vi "stop watch (1).vi"() -> ()   [LabVIEW 2016]
panel:
  out "start time":timestamp
  out "Started":bool
  in  "OK Button":bool
  out "Elapsed time (seconds)":dbl
  in  "stop":bool
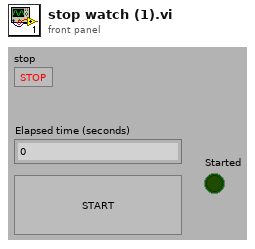
[diagram p1: front panel]
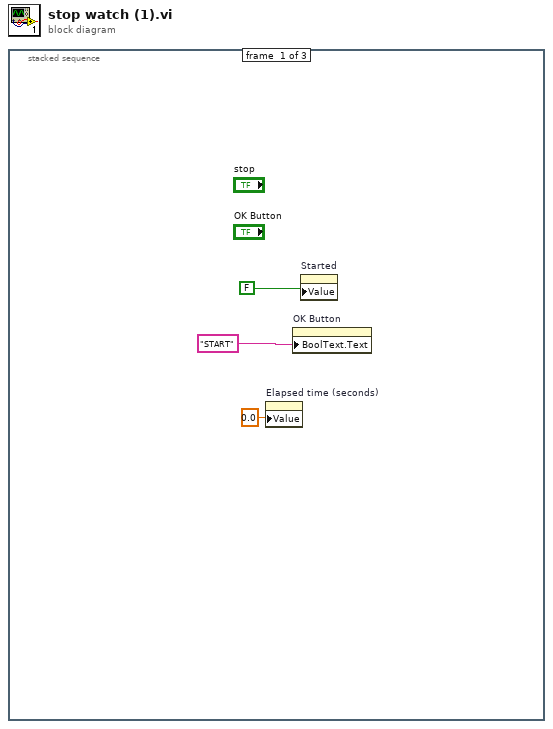
[diagram p0: block diagram]
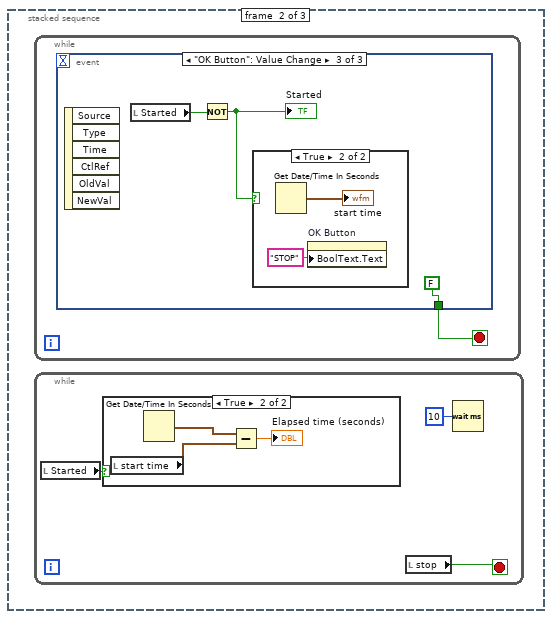
[diagram p2: hidden frame]
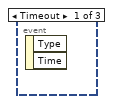
[diagram p4: hidden frame]
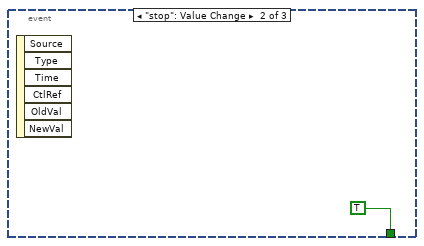
[diagram p5: hidden frame]
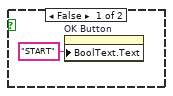
[diagram p6: hidden frame]
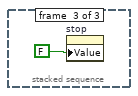
[diagram p7: hidden frame]
diagram:
  n1 = stacked-sequence {
    frame #0 {
      n2 = property on="Elapsed time (seconds)" class="DigNum (strict)"("Value"=0.0 ("Elapsed time (seconds)")) -> ()  [unwired: 2 in, 2 out]
      n3 = property on="OK Button" class="Bool"("BoolText.Text"="START" ("Caption.Text")) -> ()  [unwired: 2 in, 2 out]
      n4 = property on="Started" class="Bool (strict)"("Value"=FALSE ("Started")) -> ()  [unwired: 2 in, 2 out]
    }
    frame #1 {
      n5 = while {
        stop <- w10 stop-if-true
        n6 = event shown="[2] \"OK Button\": Value Change" {
          selector: _ -> [_ _ _]
          dyn-events: _ -> [_ _ _]
          timeout: _ -> [_ _ _]
          tunnel: [_ TRUE FALSE] -> w10
          event Timeout {
            n7 = event-data() -> ()  [unwired: 1 in, 2 out]
          }
          event "stop": Value Change {
            n8 = event-data() -> ()  [unwired: 1 in, 6 out]
          }
          event "OK Button": Value Change {
            n9 = event-data() -> ()  [unwired: 1 in, 6 out]
            n10 = local read "Started"() -> (w14:bool)
            n11 = Not(x=w14) -> (.not. x?=w12:bool)
            "Started" <- w12
            n12 = case shown="True" w12 {
              frame False {
                n13 = property on="OK Button" class="Bool"("BoolText.Text"="START" ("Caption.Text")) -> ()  [unwired: 2 in, 2 out]
              }
              frame True {
                n14 = Get Date/Time In Seconds() -> (seconds since 1Jan1904=→"start time":timestamp)
                n15 = property on="OK Button" class="Bool"("BoolText.Text"="STOP" ("Caption.Text")) -> ()  [unwired: 2 in, 2 out]
              }
            }
          }
        }
      }
      n16 = while {
        stop <- w4 stop-if-true
        n17 = local read "Started"() -> (w5:bool)
        n18 = case shown="True" w5 {
          frame False {
            # "do nothing"
          }
          frame True {
            n19 = local read "start time"() -> (w9:timestamp)
            n20 = Get Date/Time In Seconds() -> (seconds since 1Jan1904=w8:timestamp)
            n21 = Subtract(x=w8, y=w9) -> (x-y=→"Elapsed time (seconds)":dbl)
          }
        }
        n22 = local read "stop"() -> (w4:bool)
        n23 = Wait (ms)(milliseconds to wait=u32 10) -> ()  [unwired: 1 out]
      }
    }
    frame #2 {
      n24 = property on="stop" class="Bool (strict)"("Value"=FALSE ("stop")) -> ()  [unwired: 2 in, 2 out]
    }
  }
